vi "FileSyncLoop.vi"(5 "Name(FileSync)":string="FileSync", 7 "Protocol.lvclass":refnum<class "Protocol.lvclass">, 8 "error in":errorcluster, 11 "IniConfigFilePath":path) -> (0 "error out":errorcluster)   [LabVIEW 2014, in "FileSync -- Base.lvlib"]
uses:
  FileSync -- Base.lvlib
  Protocol/Protocol.lvclass
  Def-FileSyncConfig.ctl
  <userlib>/_NEVSTOP/JKI State Machine++/_Polymophic/Add State(s) to Queue By BOOL(Element).vi
  Global - FileSync.vi
  <userlib>/_OpenG.lib/file/file.llb/Compare Two Paths - Scalar__ogtk.vi
  ProtocolConfig/ProtocolConfig.lvclass
  <vilib>/Utility/config.llb/NI_LVConfig.lvlib
  <userlib>/_NEVSTOP/JKI State Machine++/JKI State Machine++.lvlib
panel:
  in  "Status":i32[](listbox)
  out "Statusbar":string
  out "Connected":bool
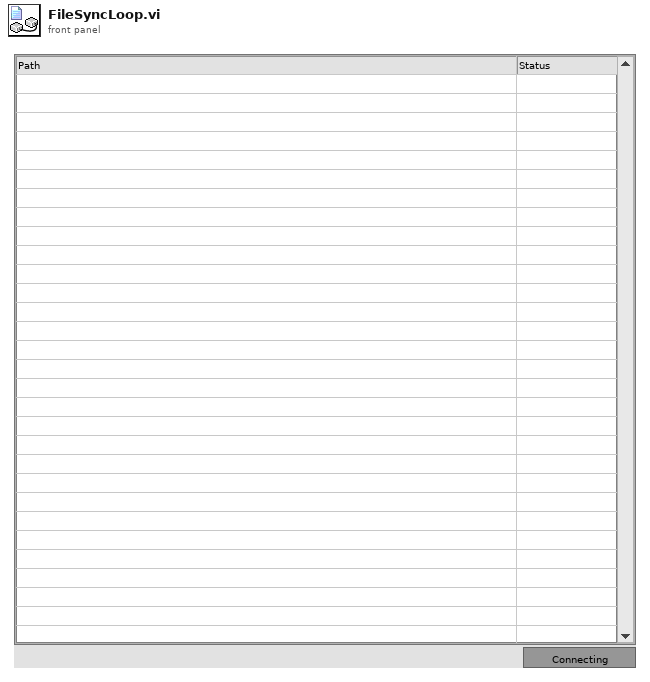
[diagram p1: front panel]
types:
  T1 = enum32{"Invalid", "Standard", "Closed", "Hidden", "Minimized", "Maximized"}
  T2 = enum32{"invalid app kind", "Development System", "Run Time System", "Student Edition", "Embedded LabVIEW", "Evaluation", "Custom"}
  T3 = typedef "FileSync -- Base.lvlib/Def-FileSyncConfig.ctl" = cluster{"Enable":bool, "DataFolder":path, "BackupFolder":path}
  T4 = cluster{"Core":cluster{"Current VI Reference":refnum<vi>, "Close Panel on Exit?":bool}, "FileSync Configuration":T3, "FileSync Status":cluster{"Connected":bool}, "Upload List":path[], "Status":refnum<vi>, "Temp:UploadingFile":path}
  T5 = cluster{"Current VI Reference":refnum<vi>, "Close Panel on Exit?":bool}
  T6 = typedef "NI_LVConfig.lvlib/Config Data RefNum.ctl" = refnum<k1>
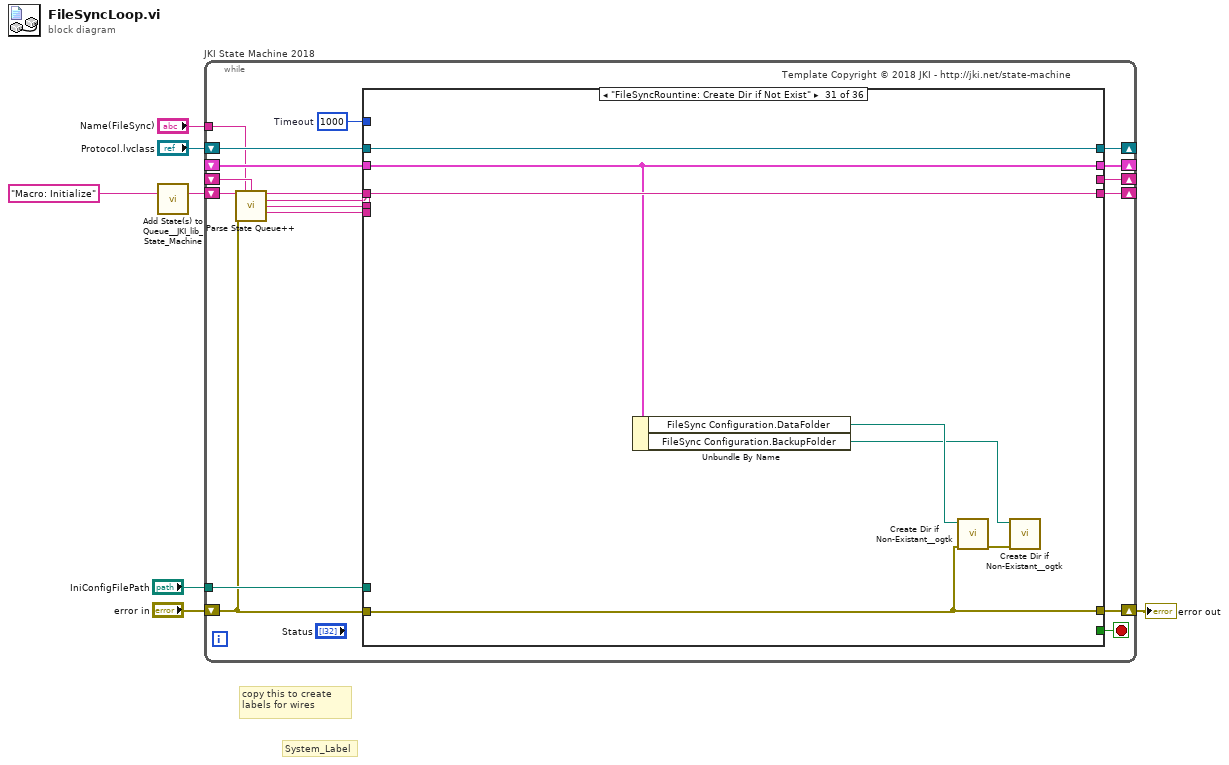
[diagram p0: block diagram]
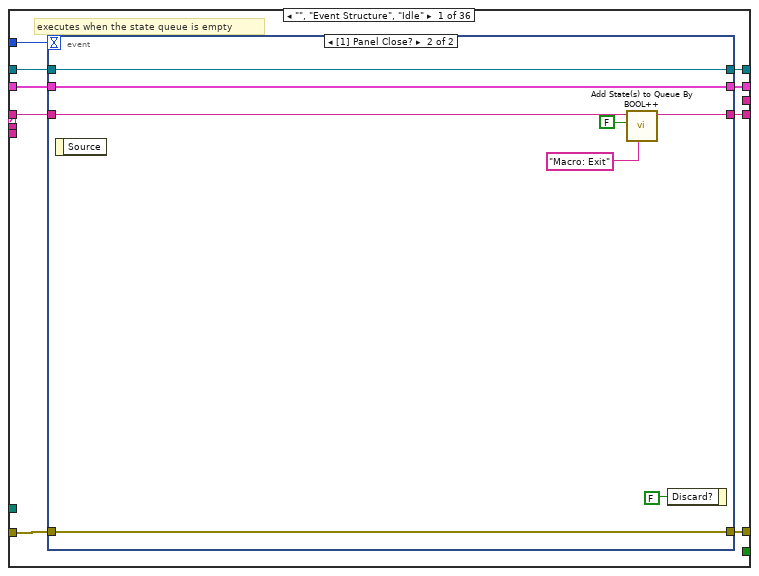
[diagram p2: hidden frame]
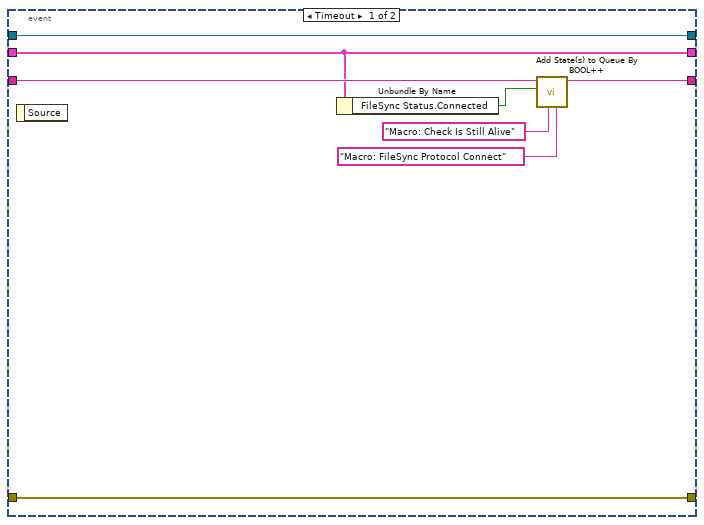
[diagram p3: hidden frame]
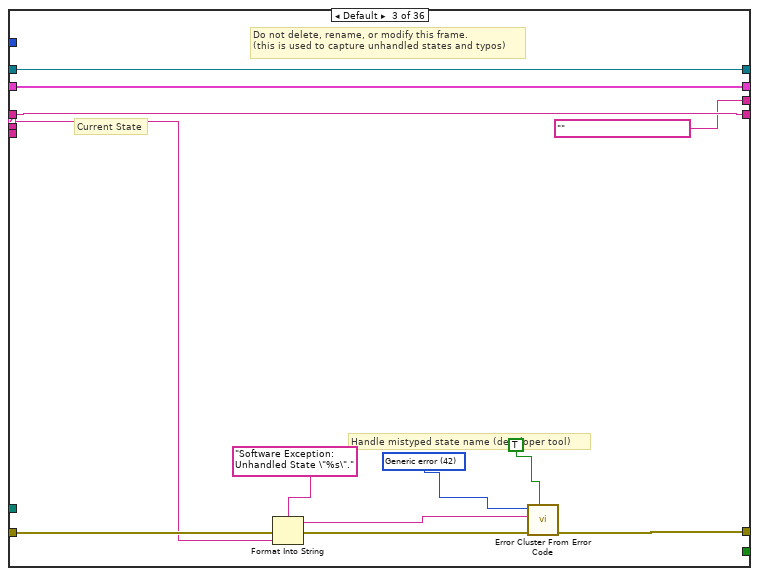
[diagram p5: hidden frame]
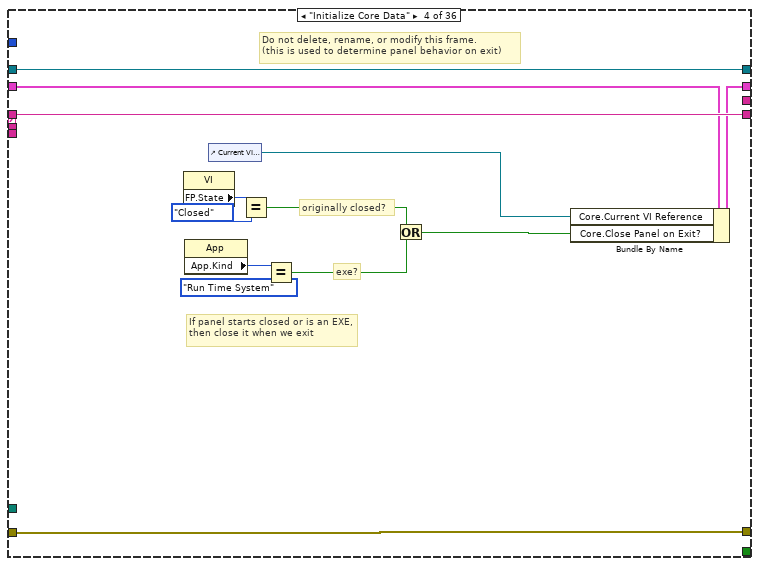
[diagram p6: hidden frame]
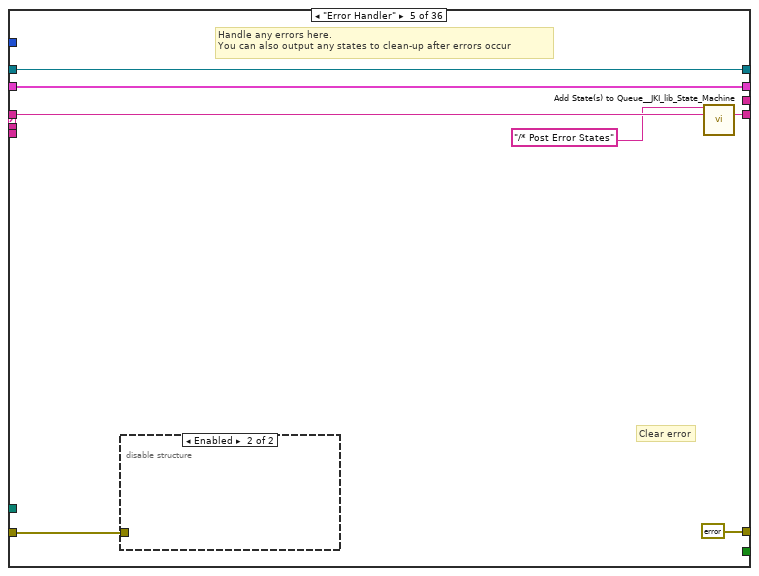
[diagram p7: hidden frame]
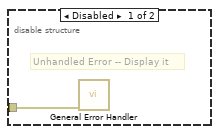
[diagram p8: hidden frame]
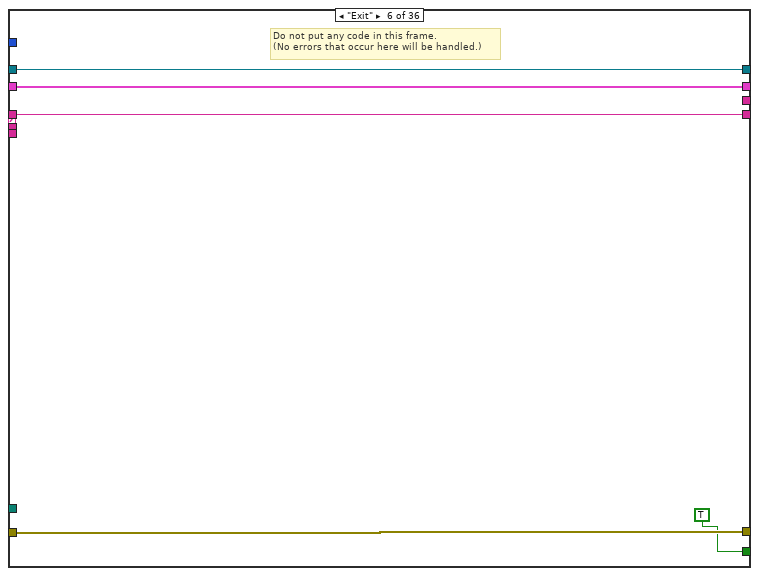
[diagram p9: hidden frame]
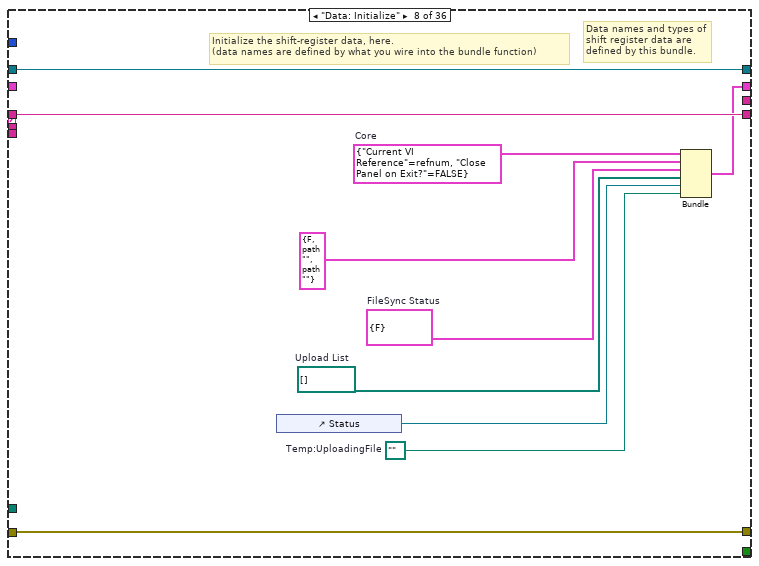
[diagram p11: hidden frame]
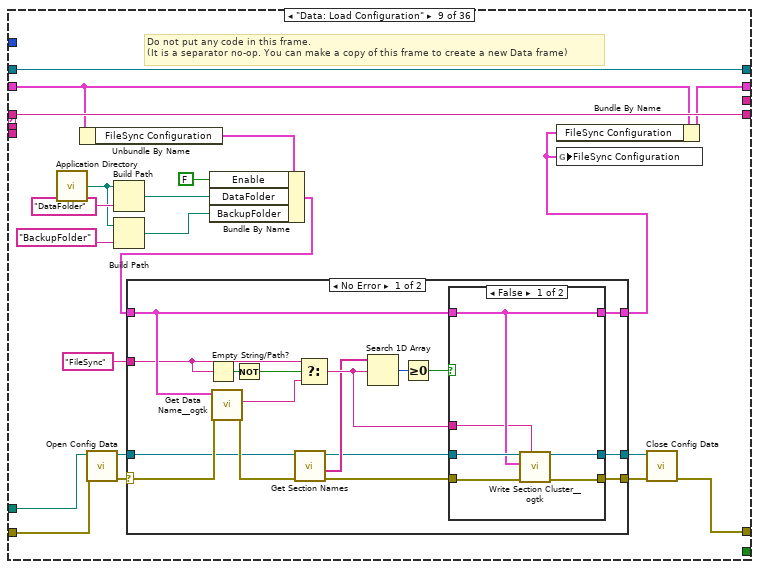
[diagram p12: hidden frame]
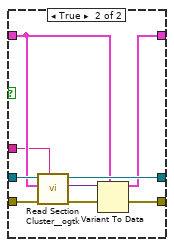
[diagram p13: hidden frame]
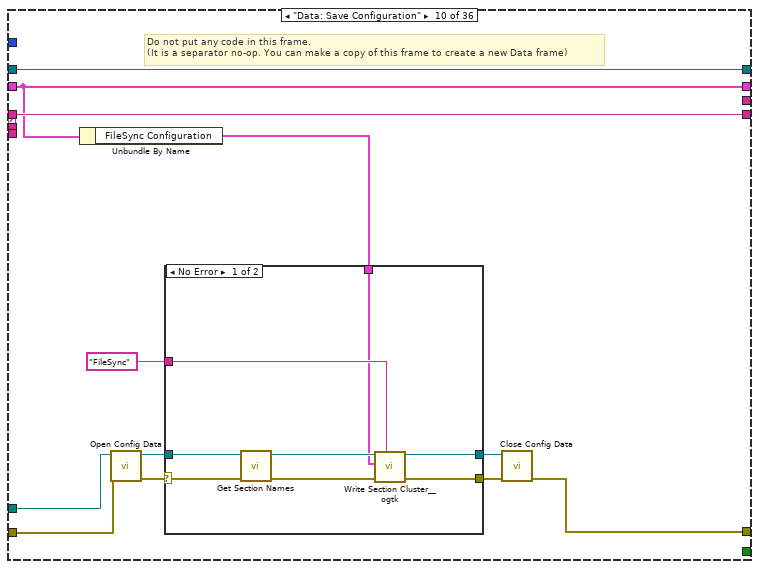
[diagram p15: hidden frame]
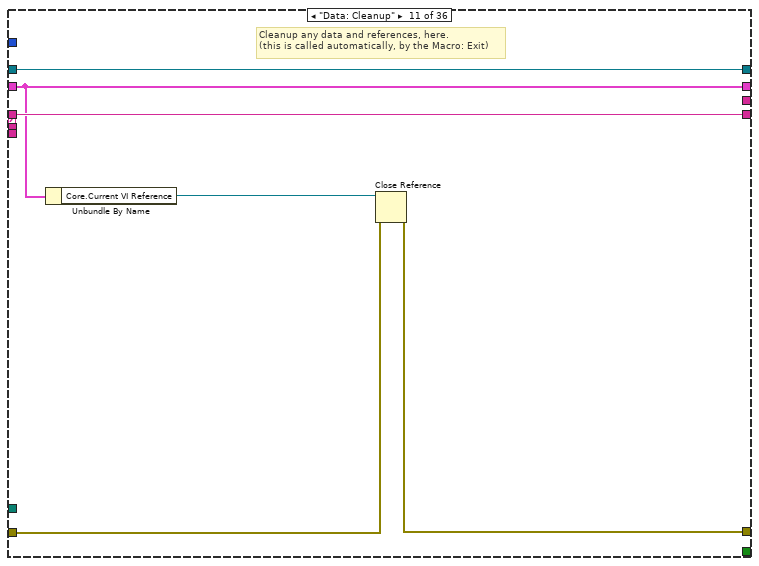
[diagram p17: hidden frame]
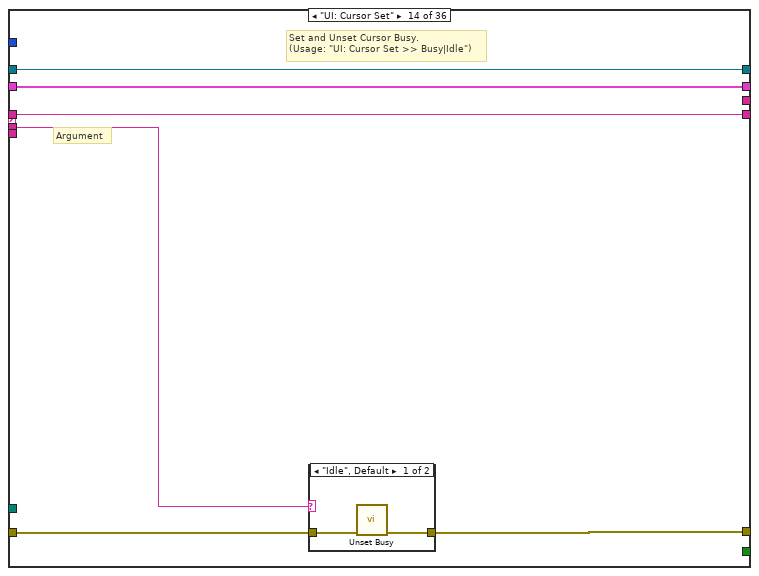
[diagram p20: hidden frame]
diagram:
  # "copy this to create labels for wires"
  # "System_Label"
  n1 = call <vilib>:"Add State(s) to Queue__JKI_lib_State_Machine.vi"("State(s) in (\"\")"="Macro: Initialize") -> ("States Out"=w7:string)  [unwired: 14 in]
  n2 = while "JKI State Machine 2018" {
    shift-right: [w22] -> _
    shift-left: _ -> [w21]
    shift-right: [w25] -> w4
    shift-left: "error in" -> [w15]
    shift-right: [w24] -> _
    shift-left: w7 -> [w16]
    shift-right: [w18] -> _
    shift-left: "Protocol.lvclass" -> [w19]
    tunnel: "IniConfigFilePath" -> [w17]
    shift-right: [w10] -> _
    shift-left: _ -> [w11]
    tunnel: "Name(FileSync)" -> [w9]
    stop <- w23 stop-if-true
    w20 = 1000  # Timeout
    # "Template Copyright © 2018 JKI - http://jki.net/state-machine"
    n3 = call <userlib>:"Parse State Queue++.vi"("State Queue"=w16, "Name(\"\" to use uuid)"=w9, "Response Arguments"=w11, "Error In (no error)"=w15) -> ("Remaining States"=w14:string, "Current State"=w12:string, "Arguments"=w13:string, "Argument - State"=w8:string)  [unwired: 6 in, 2 out]
    n4 = case shown="\"FileSyncRountine: Create Dir if Not Exist\"" w12 {
      selector: w12 -> [_ _ w57 _ _ _ _ _ _ _ _ _ _ _ _ _ _ _ _ _ _ _ _ _ _ _ _ _ _ _ _ _ _ _ _ _]
      tunnel: w14 -> [w34 w54 w60 w79 w86 w92 w96 w106 w127 w174 w190 w194 w198 w204 w215 w292 w296 w302 w306 w313 w319 w326 w341 w345 w352 w360 w371 w380 w386 w390 w397 w405 w422 w431 w441 w471]
      tunnel: w13 -> [_ _ _ _ _ _ _ _ _ _ _ _ _ w200 w210 _ _ _ _ _ _ _ _ _ _ _ _ _ _ _ _ _ _ w430 w434 w465]
      tunnel: w21 -> [w32 w52 w59 w73 w83 w91 w94 _ w118 w166 w186 w192 w197 w203 w212 w285 w294 w299 w304 w311 w317 w324 w338 w343 w351 w359 w362 w379 w385 w388 w394 w403 w418 w425 w438 w467]
      tunnel: [w31 w53 w62 w77 errorcluster {"status"=FALSE, "code"=0, "source"=""} ("error out") w90 w95 w104 w117 w165 w187 w193 w196 w201 w213 w290 w295 w300 w308 w315 w321 w328 w339 w344 w349 w355 w368 w377 w383 w389 w391 w401 w420 w427 w435 w468] -> w25
      tunnel: w15 -> [w30 w53 w61 w77 w82 w90 w95 w104 w116 w164 w188 w193 w196 w202 w214 w290 w295 w300 w308 w315 w321 w328 w339 w344 w350 w356 w369 w378 w384 w389 w391 w400 w420 w428 w439 w469]
      tunnel: [w33 w54 w60 w79 w85 w92 w96 w106 w127 w174 w190 w194 w198 w204 w215 w292 w296 w301 w307 w314 w320 w327 w340 w345 w352 w360 w370 w380 w386 w390 w397 w405 w421 w431 w441 w471] -> w24
      tunnel: [_ _ _ _ _ TRUE _ _ _ _ _ _ _ _ _ _ _ _ _ _ _ _ _ _ _ _ _ _ _ _ _ _ _ _ _ _] -> w23
      tunnel: [w29 w52 w59 w78 w83 w91 w94 w105 w119 w166 w186 w192 w197 w203 w212 w285 w294 w299 w304 w311 w317 w324 w338 w343 w351 w354 w362 w374 w385 w388 w394 w399 w417 w425 w438 w467] -> w22
      tunnel: w20 -> [w28 _ _ _ _ _ _ _ _ _ _ _ _ _ _ _ _ _ _ _ _ _ _ _ _ _ _ _ _ _ _ _ _ _ _ _]
      tunnel: w19 -> [w27 w51 w56 w67 w80 w88 w93 w102 w126 w173 w185 w191 w195 w199 w209 w291 w293 w297 w309 w316 w322 w329 w331 w342 w348 w358 w367 w376 w382 w387 w396 w404 w419 w423 w440 w470]
      tunnel: [w26 w51 w56 w67 w80 w88 w93 w102 w126 w173 w185 w191 w195 w199 w209 w289 w293 w297 w309 w316 w322 w329 w331 w342 w347 w357 w366 w375 w381 w387 w396 w404 w419 w429 w440 w470] -> w18
      tunnel: w17 -> [_ _ _ _ _ _ _ _ w120 w167 _ _ _ _ _ _ _ _ _ _ _ _ _ _ w346 _ _ _ _ _ _ _ _ _ _ _]
      tunnel: [_ _ "" ("message") _ _ _ _ _ _ _ _ _ _ _ _ _ _ _ _ _ _ _ _ _ _ _ _ _ _ _ _ _ _ _ _ _] -> w10
      tunnel: w8 -> [_ _ _ _ _ _ _ _ _ _ _ _ _ _ _ _ _ _ _ _ _ _ _ _ _ _ _ _ _ _ _ _ _ _ _ _]
      frame "", "Event Structure", "Idle" {
        # "executes when the state queue is empty"
        n5 = event shown="[1] Panel Close?" {
          selector: _ -> [_ _]
          dyn-events: _ -> [_ _]
          timeout: w28 -> [_ _]
          tunnel: w34 -> [w42 w46]
          tunnel: [w36 w50] -> w33
          tunnel: w32 -> [w39 w48]
          tunnel: [w41 w49] -> w31
          tunnel: w30 -> [w41 w49]
          tunnel: [w39 w48] -> w29
          tunnel: w27 -> [w40 w47]
          tunnel: [w40 w47] -> w26
          event Timeout {
            n6 = event-data() -> ()  [unwired: 1 in, 1 out]
            n7 = Unbundle By Name(w39) -> ("FileSync Status.Connected"=w35:bool)
            n8 = call-poly <userlib>:"Add State(s) to Queue By BOOL++.vi"("False(Empty)"="Macro: FileSync Protocol Connect" ("State(s) in Front (\"\")"), "TRUE(Empty)"="Macro: Check Is Still Alive" ("State(s) in Front (\"\")"), "Bool"=w35, "Remaining States"=w42) -> ("States Out"=w36:string)  [unwired: 7 in]
          }
          event Panel Close? {
            n9 = event-data() -> ()  [unwired: 1 in, 1 out]
            n10 = call-poly <userlib>:"Add State(s) to Queue By BOOL++.vi"("TRUE(Empty)"="Macro: Exit", "Bool"=FALSE, "Remaining States"=w46) -> ("States Out"=w50:string)  [unwired: 8 in]
            n11 = event-data("Discard?"=FALSE) -> ()  [unwired: 1 in, 1 out]
          }
        }
      }
      frame "---------- Core ----------" {
        # "Do not put any code in this frame.\n(it is a separator no-op)"
      }
      frame Default {
        w65 = 42 items=["No error", "Argument error", "Memory is full", "Out of zone", "End of file", "File already open", "Generic file I/O error", "File not found", "File permission error", "Disk is full", "Duplicate path", "Too many files open", "System feature not enabled", "Resource file not found", "Cannot add resource", "Resource not found", "Image not found", "Image memory error", "Pen does not exist", "Config type invalid", "Config token not found", "Config parse error", "Config memory error", "Bad external code format", "Bad external code offset", "External code not present", "Null window", "Destroy window error", "Null menu", "Print aborted", "Bad print record", "Print driver error", "Windows error during printing", "Memory error during printing", "Print dialog error", "Generic print error", "Invalid device refnum", "Device not found", "Device parameter error", "Device unit error", "Cannot open device", "Device call aborted", "Generic error", "Cancelled by user", "Object ID too low", "Object ID too high", "Object not in heap", "Unknown heap", "Unknown object (invalid DefProc)", "Unknown object (DefProc not in table)", "Message out of range", "Invalid (null) method", "Unknown message", "Manager call not supported", "Bad address", "Network operation in progress", "Network operation timed out", "Connection is busy", "Network attribute not supported", "Network error", "Address in use", "System out of memory", "Connection aborted", "Connection refused", "Not connected", "Already connected", "Connection closed", "Initialization error (interapplication manager)", "Bad occurrence", "Wait on unbound occurrence handler", "Occurrence queue overflow", "Datalog type conflict", "Unused", "Unrecognized type (interapplication manager)", "Memory corrupt", "Failed to make temporary DLL", "Old CIN version", "Drag socket not found", "Failed to load drop-object", "Failed to register OLE object", "Failed to release OLE object", "Format specifier type mismatch", "Unknown format specifier", "Too few format specifiers", "Too many format specifiers", "Scan failed", "Newer CIN version", "Error converting to variant", "Runtime menu error", "Password tampered", "Variant attribute not found", "Incompatible variant data type", "Event data is not available", "Event Store is not present", "Occurrence is not found", "Event Queue is not created", "Event info is not available", "Refnum passed is NULL", "Error retrieving Class GUID", "Error retrieving CoClass GUID", "Error retrieving TypeLib GUID.", "Bad built application magic bytes.", "Specific driver is different from the specific driver associated with the Logical Name.", "There is no session opened to the class driver.", "Max Error", "MAX - Error with config objects", "MAX - Error loading configuration", "MAX - Group not supported"]
        # "Current State"
        # "Do not delete, rename, or modify this frame.\n(this is used to capture unhandled states and typos)"
        # "Handle mistyped state name (developer tool)"
        n12 = Format Into String(format string="Software Exception: Unhandled State \"%s\"." ("message"), error in=w61, w57) -> (resulting string=w64:string, error out=w63:errorcluster)  [unwired: 1 in]
        n13 = call <vilib>:"Error Cluster From Error Code.vi"("show call chain? (False)"=TRUE, "error in (no error)"=w63, "error message (\"\")"=w64, "error code (0)"=w65) -> ("error out"=w62:errorcluster)  [unwired: 5 in]
      }
      frame "Initialize Core Data" {
        # "Do not delete, rename, or modify this frame.\n(this is used to determine panel behavior on exit)"
        # "originally closed?"
        # "exe?"
        # "If panel starts closed or is an EXE, then close it when we exit"
        n14 = property class="VI"() -> ("FP.State"=w70:T1)  [unwired: 2 in, 2 out]
        n15 = property class="App"() -> ("App.Kind"=w76:T2)  [unwired: 2 in, 2 out]
        n16 = control-ref of="Current VI Reference"() -> (w71:refnum<vi>)
        n17 = Equal?(x=w70, y=T1."Closed" ("Front Panel Window:State")) -> (x = y?=w68:bool)
        n18 = Equal?(x=w76, y=T2."Run Time System" ("Application:Kind")) -> (x = y?=w74:bool)
        n19 = Or(x=w68, y=w74) -> (x .or. y?=w72:bool)
        n20 = Bundle By Name(cluster=w73, "Core.Current VI Reference"=w71, "Core.Close Panel on Exit?"=w72) -> (w78:T4)
      }
      frame "Error Handler" {
        # "Handle any errors here.\nYou can also output any states to clean-up after errors occur"
        # "Clear error"
        n21 = disable-structure shown="Enabled" {
          disable-tunnel: w82 -> [w87 _]
          frame Disabled {
            # "Unhandled Error -- Display it"
            n22 = call <vilib>:"General Error Handler.vi"("error in (no error)"=w87) -> ()  [unwired: 10 in, 5 out]
          }
          frame Enabled {
          }
        }
        n23 = call <vilib>:"Add State(s) to Queue__JKI_lib_State_Machine.vi"("State(s) in Front (\"\")"="/* Post Error States", "State(s) in (\"\")"=w86) -> ("States Out"=w85:string)  [unwired: 13 in]
      }
      frame "Exit" {
        # "Do not put any code in this frame.\n(No errors that occur here will be handled.)"
      }
      frame "---------- Data ----------" {
        # "Do not put any code in this frame.\n(It is a separator no-op. You can make a copy of this frame to create a new Data frame)"
      }
      frame "Data: Initialize" {
        w97 = path ""  # Temp:UploadingFile
        w98 = path[] []  # Upload List
        w99 = cluster{"Connected":bool} {"Connected"=FALSE}  # FileSync Status
        w103 = T5 {"Current VI Reference"=refnum, "Close Panel on Exit?"=FALSE}  # Core
        # "Data names and types of shift register data are defined by this bundle."
        # "Initialize the shift-register data, here.\n(data names are defined by what you wire into the bundle function)"
        n24 = control-ref of="Status"() -> (w101:refnum<vi>)
        n25 = Bundle("Core"=w103, "FileSync Configuration"=T3 {"Enable"=FALSE, "DataFolder"=path "", "BackupFolder"=path ""}, "FileSync Status"=w99, "Upload List"=w98, "Status"=w101, "Temp:UploadingFile"=w97) -> (w105:T4)  [unwired: 1 in]
      }
      frame "Data: Load Configuration" {
        # "Do not put any code in this frame.\n(It is a separator no-op. You can make a copy of this frame to create a new Data frame)"
        n26 = call <vilib>:"Application Directory.vi"() -> ("Application Directory"=w110:path)
        n27 = Unbundle By Name(w118) -> ("FileSync Configuration"=w115:T3)
        n28 = call <vilib>:"Open Config Data.vi"("error in (no error)"=w116, "configuration file path"=w120) -> ("error out"=w124:errorcluster, "refnum"=w125:T6)  [unwired: 7 in, 1 out]
        n29 = Build Path(base path=w110, name or relative path="DataFolder") -> (appended path=w108:path)
        n30 = Build Path(base path=w110, name or relative path="BackupFolder") -> (appended path=w109:path)
        n31 = Bundle By Name(cluster=w115, "Enable"=FALSE, "DataFolder"=w108, "BackupFolder"=w109) -> (w113:T3)
        n32 = case shown="No Error" w124 {
          selector: w124 -> [w142 w160]
          tunnel: w113 -> [w141 w162]
          tunnel: "FileSync" ("section") -> [w139 _]
          tunnel: w125 -> [w131 w161]
          tunnel: [w130 w160] -> w122
          tunnel: [w129 w161] -> w123
          tunnel: [w128 w162] -> w107
          frame No Error {
            n33 = Empty String/Path?(string/path=w139) -> (empty?=w137:bool)
            n34 = call <userlib>:"Get Data Name__ogtk.vi"("error in (no error)"=w142, "Data"=w141) -> ("error out"=w143:errorcluster, "Data Name"=w140:string)  [unwired: 7 in, 1 out]
            n35 = Not(x=w137) -> (.not. x?=w138:bool)
            n36 = call <vilib>:"Get Section Names.vi"("error in (no error)"=w143, "refnum"=w131) -> ("error out"=w133:errorcluster, "section names"=w134:string[], "refnum out"=w132:T6)  [unwired: 7 in]
            n37 = Select(t=w139, s=w138, f=w140) -> (s? t:f=w144:string)
            n38 = Search 1D Array(1D array=w134, element=w144) -> (index of element=w135:i32)  [unwired: 1 in]
            n39 = Greater Or Equal To 0?(x=w135) -> (x >= 0?=w136:bool)
            n40 = case shown="False" w136 {
              tunnel: w132 -> [w150 w159]
              tunnel: [w149 w158] -> w129
              tunnel: w133 -> [w147 w157]
              tunnel: [w148 w155] -> w130
              tunnel: w141 -> [w146 w153]
              tunnel: [w146 w154] -> w128
              tunnel: w144 -> [w145 w152]
              frame False {
                n41 = call <userlib>:"Write Section Cluster__ogtk.vi"("section (optional)"=w145, "error in (no error)"=w147, "Section Formatted Cluster"=w146, "refnum"=w150) -> ("error out"=w148:errorcluster, "dup refnum"=w149:T6)  [unwired: 6 in]
              }
              frame True {
                n42 = call <userlib>:"Read Section Cluster__ogtk.vi"("section (optional)"=w152, "error in (no error)"=w157, "Section Formatted Cluster Type"=w153, "refnum"=w159) -> ("error out"=w156:errorcluster, "Section Formatted Cluster"=w151:variant, "dup refnum"=w158:T6)  [unwired: 3 in, 2 out]
                n43 = Variant To Data(error in=w156, type=w153, Variant=w151) -> (data=w154:T3, error out=w155:errorcluster)
              }
            }
          }
          frame Error {
          }
        }
        n44 = Bundle By Name(cluster=w118, "FileSync Configuration"=w107) -> (w119:T4)
        n45 = global write "Global - FileSync.vi" "FileSync Configuration"(w107) -> ()
        n46 = call <vilib>:"Close Config Data.vi"("error in (no error)"=w122, "refnum"=w123) -> ("error out"=w117:errorcluster)  [unwired: 8 in, 1 out]
      }
      frame "Data: Save Configuration" {
        # "Do not put any code in this frame.\n(It is a separator no-op. You can make a copy of this frame to create a new Data frame)"
        n47 = Unbundle By Name(w166) -> ("FileSync Configuration"=w163:T3)
        n48 = call <vilib>:"Open Config Data.vi"("error in (no error)"=w164, "configuration file path"=w167) -> ("error out"=w171:errorcluster, "refnum"=w172:T6)  [unwired: 7 in, 1 out]
        n49 = case shown="No Error" w171 {
          selector: w171 -> [w175 w183]
          tunnel: "FileSync" ("section") -> [w177 _]
          tunnel: w172 -> [w180 w184]
          tunnel: [w179 w183] -> w169
          tunnel: [w178 w184] -> w170
          tunnel: w163 -> [w176 _]
          frame No Error {
            n50 = call <vilib>:"Get Section Names.vi"("error in (no error)"=w175, "refnum"=w180) -> ("error out"=w182:errorcluster, "refnum out"=w181:T6)  [unwired: 7 in, 1 out]
            n51 = call <userlib>:"Write Section Cluster__ogtk.vi"("section (optional)"=w177, "error in (no error)"=w182, "Section Formatted Cluster"=w176, "refnum"=w181) -> ("error out"=w179:errorcluster, "dup refnum"=w178:T6)  [unwired: 6 in]
          }
          frame Error {
          }
        }
        n52 = call <vilib>:"Close Config Data.vi"("error in (no error)"=w169, "refnum"=w170) -> ("error out"=w165:errorcluster)  [unwired: 8 in, 1 out]
      }
      frame "Data: Cleanup" {
        # "Cleanup any data and references, here.\n(this is called automatically, by the Macro: Exit)"
        n53 = Unbundle By Name(w186) -> ("Core.Current VI Reference"=w189:refnum<vi>)
        n54 = Close Reference(reference=w189, error in (no error)=w188) -> (error out=w187:errorcluster)
      }
      frame "---------- UI ----------" {
        # "Do not put any code in this frame.\n(It is a separator no-op. You can make a copy of this frame to create a new UI frame)"
      }
      frame "UI: Initialize" {
      }
      frame "UI: Cursor Set" {
        # "Argument"
        # "Set and Unset Cursor Busy.\n(Usage: \"UI: Cursor Set >> Busy|Idle\")"
        n55 = case shown="\"Idle\", Default" w200 {
          tunnel: w202 -> [w206 w208]
          tunnel: [w205 w207] -> w201
          frame "Idle", Default {
            n56 = call <vilib>:"Unset Busy.vi"("error in (no error)"=w206) -> ("error out"=w205:errorcluster)  [unwired: 10 in]
          }
          frame "Busy" {
            n57 = call <vilib>:"Set Busy.vi"("error in (no error)"=w208) -> ("error out"=w207:errorcluster)  [unwired: 9 in, 1 out]
          }
        }
      }
      frame "UI: Front Panel State" {
        # "Argument"
        # "Set Front Panel Open or Closed\n(Usage: \"UI: Front Panel State >> Open|Close\")"
        n58 = Unbundle By Name(w212) -> ("Core.Current VI Reference"=w211:refnum<vi>)
        n59 = case shown="\"Open\", \"Standard\", Default" w210 {
          tunnel: w214 -> [w221 w236 w247 w260 w273]
          tunnel: [w223 w237 w249 w262 w275] -> w213
          tunnel: w211 -> [w222 w234 w248 w261 w274]
          frame "Open", "Standard", Default {
            w216 = T1."Standard" ("State")
            n60 = property class="VI"(reference=w222, error in=w221) -> (reference out=w219:refnum<vi>, error out=w220:errorcluster, "FP.State"=w218:T1)
            n61 = Not Equal?(x=w218, y=w216) -> (x != y?=w217:bool)
            n62 = case shown="True" w217 {
              tunnel: [w227 w229] -> w223
              tunnel: w220 -> [w226 w229]
              tunnel: w219 -> [w225 _]
              tunnel: w216 -> [w224 _]
              frame True {
                n63 = invoke class="VI" method="FP.Open"(reference=w225, error in=w226, "Activate"=TRUE, "State"=w224) -> (error out=w227:errorcluster)  [unwired: 1 in, 4 out]
              }
              frame False {
              }
            }
          }
          frame "Close", "Closed" {
            n64 = property class="VI"(reference=w234, error in=w236) -> (reference out=w233:refnum<vi>, error out=w235:errorcluster, "FP.State"=w231:T1)
            n65 = Not Equal?(x=w231, y=T1."Closed" ("Front Panel Window:State")) -> (x != y?=w230:bool)
            n66 = case shown="True" w230 {
              tunnel: [w238 w241] -> w237
              tunnel: w235 -> [w238 w240]
              tunnel: w233 -> [_ w239]
              frame False {
              }
              frame True {
                n67 = invoke class="VI" method="FP.Close"(reference=w239, error in=w240) -> (error out=w241:errorcluster)  [unwired: 1 in, 2 out]
              }
            }
          }
          frame "Hidden", "Hide" {
            w242 = T1."Hidden" ("State")
            n68 = property class="VI"(reference=w248, error in=w247) -> (reference out=w245:refnum<vi>, error out=w246:errorcluster, "FP.State"=w244:T1)
            n69 = Not Equal?(x=w244, y=w242) -> (x != y?=w243:bool)
            n70 = case shown="True" w243 {
              tunnel: [w253 w254] -> w249
              tunnel: w246 -> [w252 w254]
              tunnel: w245 -> [w251 _]
              tunnel: w242 -> [w250 _]
              frame True {
                n71 = invoke class="VI" method="FP.Open"(reference=w251, error in=w252, "State"=w250) -> (error out=w253:errorcluster)  [unwired: 2 in, 4 out]
              }
              frame False {
              }
            }
          }
          frame "Minimize", "Minimized" {
            w255 = T1."Minimized" ("State")
            n72 = property class="VI"(reference=w261, error in=w260) -> (reference out=w258:refnum<vi>, error out=w259:errorcluster, "FP.State"=w257:T1)
            n73 = Not Equal?(x=w257, y=w255) -> (x != y?=w256:bool)
            n74 = case shown="True" w256 {
              tunnel: [w266 w267] -> w262
              tunnel: w259 -> [w265 w267]
              tunnel: w258 -> [w264 _]
              tunnel: w255 -> [w263 _]
              frame True {
                n75 = invoke class="VI" method="FP.Open"(reference=w264, error in=w265, "State"=w263) -> (error out=w266:errorcluster)  [unwired: 2 in, 4 out]
              }
              frame False {
              }
            }
          }
          frame "Maximize", "Maximized" {
            w268 = T1."Maximized" ("State")
            n76 = property class="VI"(reference=w274, error in=w273) -> (reference out=w271:refnum<vi>, error out=w272:errorcluster, "FP.State"=w270:T1)
            n77 = Not Equal?(x=w270, y=w268) -> (x != y?=w269:bool)
            n78 = case shown="True" w269 {
              tunnel: [w279 w280] -> w275
              tunnel: w272 -> [w278 w280]
              tunnel: w271 -> [w277 _]
              tunnel: w268 -> [w276 _]
              frame True {
                n79 = invoke class="VI" method="FP.Open"(reference=w277, error in=w278, "State"=w276) -> (error out=w279:errorcluster)  [unwired: 2 in, 4 out]
              }
              frame False {
              }
            }
          }
        }
      }
      frame "UI: Update" {
        n80 = Unbundle By Name(w285) -> ("Status"=w283:refnum<vi>, "FileSync Status.Connected"=w284:bool, "Upload List"=w282:path[], "Temp:UploadingFile"=w281:path)
        "Connected" <- w284
        n81 = property class="Protocol.lvclass"(reference=w291) -> (reference out=w289:refnum<class "Protocol.lvclass">, "Properties:ProtocolConfig.lvclass"=w288:refnum<class "ProtocolConfig.lvclass">)  [unwired: 1 in, 1 out]
        n82 = call-dynamic "FlattenToDisplayString.vi"("ProtocolConfig in"=w288) -> ("String"=→"Statusbar":string)  [unwired: 8 in, 2 out]
        n83 = call "Prepare Status Table.vi"("MulticolumnListbox in"=w283, "Temp:UploadingFile"=w281, "Upload List"=w282) -> ("Array"=w286:string[][])  [unwired: 8 in]
        n84 = global write "Global - FileSync.vi" "Connected"(w284) -> ()
        n85 = property on="Status" class="MCListbox (strict)"("ItemNames"=w286) -> ()  [unwired: 2 in, 2 out]
      }
      frame "---------- Macro ----------" {
        # "Do not put any code in this frame.\n(It is a separator no-op. You can make a copy of this frame to create a new Macro frame)"
      }
      frame "Macro: Initialize" {
        # "Initialization Macro\n(This is called once, when the VI starts)"
        n86 = call <vilib>:"Add State(s) to Queue__JKI_lib_State_Machine.vi"("State(s) in Front (\"\")"="Data: Initialize\nInitialize Core Data\nData: Load Configuration\nUI: Initialize\nUI: Update\n//UI: Front Panel State >> Open\n", "State(s) in (\"\")"=w302) -> ("States Out"=w301:string)  [unwired: 13 in]
      }
      frame "Macro: FileSync Protocol Connect" {
        n87 = Unbundle By Name(w304) -> ("FileSync Configuration.Enable"=w303:bool)
        n88 = case shown="True" w303 {
          tunnel: [_ "FileSync: Load Configuration\nFileSync: Try to Connect\nUI: Update" ("State(s) in Front (\"\")")] -> w305
          frame False {
          }
          frame True {
          }
        }
        n89 = call <vilib>:"Add State(s) to Queue__JKI_lib_State_Machine.vi"("State(s) in Front (\"\")"=w305, "State(s) in (\"\")"=w306) -> ("States Out"=w307:string)  [unwired: 13 in]
      }
      frame "Macro: Check Is Still Alive" {
        n90 = call <vilib>:"Add State(s) to Queue__JKI_lib_State_Machine.vi"("State(s) in Front (\"\")"="FileSync: Check Connection is Still Alive\nUI: Update" ("State(s) in Front (\"\")"), "State(s) in (\"\")"=w313) -> ("States Out"=w314:string)  [unwired: 13 in]
      }
      frame "Macro: FileSync Routines" {
        n91 = call <vilib>:"Add State(s) to Queue__JKI_lib_State_Machine.vi"("State(s) in Front (\"\")"="FileSyncRountine: Create Dir if Not Exist\nFileSyncRountine: List Files\nFileSyncRountine: Pick Uploading File\nUI: Update" ("State(s) in Front (\"\")"), "State(s) in (\"\")"=w319) -> ("States Out"=w320:string)  [unwired: 13 in]
      }
      frame "Macro: FileSync Protocol Disconnect" {
        n92 = Unbundle By Name(w324) -> ("FileSync Status.Connected"=w323:bool)
        n93 = case shown="True" w323 {
          tunnel: [_ "FileSync: Close Connection\nFileSync: Cleanup Protocol\nUI: Update" ("State(s) in Front (\"\")")] -> w325
          frame False {
          }
          frame True {
          }
        }
        n94 = call <vilib>:"Add State(s) to Queue__JKI_lib_State_Machine.vi"("State(s) in Front (\"\")"=w325, "State(s) in (\"\")"=w326) -> ("States Out"=w327:string)  [unwired: 13 in]
      }
      frame "Macro: Exit" {
        # "Exit Macro\n(This is called once, when the VI exits)"
        n95 = Unbundle By Name(w338) -> ("Core.Close Panel on Exit?"=w337:bool)
        n96 = Select(t="UI: Front Panel State >> Close", s=w337, f="") -> (s? t:f=w334:string)
        n97 = call <vilib>:"Add State(s) to Queue__JKI_lib_State_Machine.vi"("State(s) in (\"\")"=w334, "State(s) at Back (\"\")"="Macro: FileSync Protocol Disconnect\nData: Cleanup\nExit") -> ("States Out"=w332:string)  [unwired: 13 in]
        n98 = call <vilib>:"Add State(s) to Queue__JKI_lib_State_Machine.vi"("State(s) in Front (\"\")"=w332, "State(s) in (\"\")"=w341) -> ("States Out"=w340:string)  [unwired: 13 in]
      }
      frame "---------- FileSync ----------" {
      }
      frame "FileSync: Load Configuration" {
        n99 = call-dynamic "Initialize.vi"("error in (no error)"=w350, "Path"=w346, "Protocol in"=w348) -> ("error out"=w349:errorcluster, "Protocol out"=w347:refnum<class "Protocol.lvclass">)  [unwired: 7 in]
      }
      frame "FileSync: Try to Connect" {
        n100 = call-dynamic "Connect.vi"("error in (no error)"=w356, "Protocol in"=w358) -> ("error out"=w355:errorcluster, "Connected?"=w353:bool, "Protocol out"=w357:refnum<class "Protocol.lvclass">)  [unwired: 7 in]
        n101 = Bundle By Name(cluster=w359, "FileSync Status.Connected"=w353) -> (w354:T4)
      }
      frame "FileSync: Check Connection is Still Alive" {
        n102 = call-dynamic "Check.vi"("error in (no error)"=w369, "Protocol in"=w367) -> ("error out"=w368:errorcluster, "Still alive?"=w365:bool, "Protocol out"=w366:refnum<class "Protocol.lvclass">)  [unwired: 7 in]
        n103 = Unbundle By Name(w362) -> ("FileSync Configuration.Enable"=w361:bool)
        n104 = case shown="True" w361 {
          tunnel: [_ "Macro: FileSync Routines" ("State(s) in Front (\"\")")] -> w364
          frame False {
          }
          frame True {
          }
        }
        n105 = call-poly <userlib>:"Add State(s) to Queue By BOOL++.vi"("False(Empty)"="Macro: FileSync Protocol Disconnect" ("State(s) in Front (\"\")"), "TRUE(Empty)"=w364, "Bool"=w365, "Remaining States"=w371) -> ("States Out"=w370:string)  [unwired: 7 in]
      }
      frame "FileSync: Close Connection" {
        n106 = Bundle By Name(cluster=w379, "FileSync Status.Connected"=FALSE) -> (w374:T4)
        n107 = call-dynamic "Disconnect.vi"("error in (no error)"=w378, "Protocol in"=w376) -> ("error out"=w377:errorcluster, "Protocol out"=w375:refnum<class "Protocol.lvclass">)  [unwired: 8 in]
      }
      frame "FileSync: Cleanup Protocol" {
        n108 = call-dynamic "Cleanup.vi"("error in (no error)"=w384, "Protocol in"=w382) -> ("error out"=w383:errorcluster, "Protocol out"=w381:refnum<class "Protocol.lvclass">)  [unwired: 8 in]
      }
      frame "---------- FileSyncRountine ----------" {
      }
      frame "FileSyncRountine: Create Dir if Not Exist" {
        n109 = Unbundle By Name(w394) -> ("FileSync Configuration.DataFolder"=w393:path, "FileSync Configuration.BackupFolder"=w392:path)
        n110 = call <userlib>:"Create Dir if Non-Existant__ogtk.vi"("error in (no error)"=w391, "Directory Path"=w393) -> ("error out"=w395:errorcluster)  [unwired: 7 in, 2 out]
        n111 = call <userlib>:"Create Dir if Non-Existant__ogtk.vi"("error in (no error)"=w395, "Directory Path"=w392) -> ()  [unwired: 7 in, 3 out]
      }
      frame "FileSyncRountine: List Files" {
        n112 = Unbundle By Name(w403) -> ("FileSync Configuration.DataFolder"=w402:path)
        n113 = call <vilib>:"Recursive File List.vi"("error in (no error)"=w400, "Folder Path"=w402) -> ("error out"=w401:errorcluster, "All Files in Dir"=w398:path[])  [unwired: 5 in, 3 out]
        n114 = Bundle By Name(cluster=w403, "Upload List"=w398) -> (w399:T4)
      }
      frame "FileSyncRountine: Pick Uploading File" {
        n115 = Unbundle By Name(w418) -> ("Upload List"=w407:path[])
        n116 = Index Array(array=w407) -> (element=w406:path)  [unwired: 1 in]
        n117 = Bundle By Name(cluster=w418, "Temp:UploadingFile"=w406) -> (w417:T4)
        n118 = Path To String(path=w406) -> (string=w409:string)
        n119 = Empty String/Path?(string/path=w406) -> (empty?=w416:bool)
        n120 = call <vilib>:"Build State String with Arguments__JKI_lib_State_Machine.vi"("Arguments (\"\")"=w409, "State"="FileSyncRountine: Upload" ("False(Empty)")) -> ("State with Arguments"=w408:string)  [unwired: 4 in]
        n121 = call <vilib>:"Build State String with Arguments__JKI_lib_State_Machine.vi"("Arguments (\"\")"=w409, "State"="FileSyncRountine: Move File to Backup Folder" ("False(Empty)")) -> ("State with Arguments"=w411:string)  [unwired: 4 in]
        n122 = call <vilib>:"Build State String with Arguments__JKI_lib_State_Machine.vi"("Arguments (\"\")"=w409, "State"="FileSyncRountine: Remove Empty Container Folder" ("False(Empty)")) -> ("State with Arguments"=w412:string)  [unwired: 4 in]
        n123 = call <vilib>:"Add State(s) to Queue__JKI_lib_State_Machine.vi"("State(s) in Front (\"\")"=w408, "State(s) in (\"\")"=w411, "State(s) at Back (\"\")"=w412) -> ("States Out"=w413:string)  [unwired: 12 in]
        n124 = call-poly <userlib>:"Add State(s) to Queue By BOOL++.vi"("False(Empty)"=w413, "Bool"=w416, "Remaining States"=w422) -> ("States Out"=w421:string)  [unwired: 8 in]
      }
      frame "FileSyncRountine: Upload" {
        n125 = String To Path(string=w430) -> (path=w426:path)
        n126 = Unbundle By Name(w425) -> ("FileSync Configuration.DataFolder"=w424:path)
        n127 = call-dynamic "UploadFile.vi"("Root Path"=w424, "error in (no error)"=w428, "Path"=w426, "Protocol in"=w423) -> ("error out"=w427:errorcluster, "Protocol out"=w429:refnum<class "Protocol.lvclass">)  [unwired: 6 in]
      }
      frame "FileSyncRountine: Move File to Backup Folder" {
        n128 = Unbundle By Name(w438) -> ("FileSync Configuration.BackupFolder"=w437:path, "FileSync Configuration.DataFolder"=w436:path)  [unwired: 1 out]
        n129 = String To Path(string=w434) -> (path=w433:path)
        n130 = Empty String/Path?(string/path=w433) -> (empty?=w432:bool)
        n131 = case shown="False" w432 {
          tunnel: w439 -> [w455 w462]
          tunnel: w437 -> [w453 _]
          tunnel: w436 -> [w451 _]
          tunnel: w433 -> [w442 _]
          tunnel: [w443 w462] -> w435
          frame False {
            n132 = call-poly <userlib>:"Compare Two Paths__ogtk.vi"("path2"=w442, "path1"=w451) -> ("relative path from 1 to 2"=w454:path)  [unwired: 1 in, 2 out]
            n133 = Build Path(base path=w453, name or relative path=w454) -> (appended path=w452:path)
            n134 = call <vilib>:"Check if File or Folder Exists.vi"("error in (no error)"=w455, "path"=w452) -> ("error out"=w448:errorcluster, "file or folder exists?"=w449:bool, "dup path"=w450:path)  [unwired: 7 in]
            n135 = case shown="True" w449 {
              tunnel: w450 -> [w457 w461]
              tunnel: [w457 w460] -> w447
              tunnel: w448 -> [w456 w459]
              tunnel: [w456 w458] -> w445
              frame False {
              }
              frame True {
                n136 = Delete(path (use dialog)=w461, error in=w459) -> (deleted path=w460:path, error out=w458:errorcluster)  [unwired: 3 in, 1 out]
              }
            }
            n137 = Strip Path(path=w447) -> (stripped path=w446:path)  [unwired: 1 out]
            n138 = call <userlib>:"Create Dir if Non-Existant__ogtk.vi"("error in (no error)"=w445, "Directory Path"=w446) -> ("error out"=w444:errorcluster)  [unwired: 7 in, 2 out]
            n139 = Move(source path=w442, error in=w444, 10:w447) -> (error out=w443:errorcluster)  [unwired: 2 in, 2 out]
          }
          frame True {
          }
        }
      }
      frame "FileSyncRountine: Remove Empty Container Folder" {
        n140 = Unbundle By Name(w467) -> ("FileSync Configuration.DataFolder"=w466:path)  [unwired: 1 out]
        n141 = String To Path(string=w465) -> (path=w464:path)
        n142 = Empty String/Path?(string/path=w464) -> (empty?=w463:bool)
        n143 = case shown="False" w463 {
          tunnel: w469 -> [w475 w497]
          tunnel: [w474 w497] -> w468
          tunnel: w466 -> [w473 _]
          tunnel: w464 -> [w472 _]
          frame False {
            n144 = while {
              tunnel: w473 -> [w482]
              shift-right: [w478] -> w474
              shift-left: w475 -> [w479]
              shift-right: [w477] -> _
              shift-left: w472 -> [w483]
              stop <- w476 stop-if-true
              n145 = Strip Path(path=w483) -> (stripped path=w477:path)  [unwired: 1 out]
              n146 = List Folder(path=w477, error in=w479) -> (path out=w484:path, filenames=w490:string[], folder names=w489:string[], error out=w481:errorcluster)  [unwired: 2 in]
              n147 = Empty Array?(array=w490) -> (empty?=w488:bool)
              n148 = Empty Array?(array=w489) -> (empty?=w487:bool)
              n149 = Not Equal?(x=w482, y=w477) -> (x != y?=w485:bool)
              n150 = And(x=w488, y=w487) -> (x .and. y?=w486:bool)
              n151 = And(x=w485, y=w486) -> (x .and. y?=w480:bool)
              n152 = case shown="False" w480 {
                tunnel: w484 -> [_ w496]
                tunnel: w481 -> [w492 w495]
                tunnel: [w492 w494] -> w478
                tunnel: [TRUE FALSE] -> w476
                frame False {
                }
                frame True {
                  n153 = Delete(path (use dialog)=w496, error in=w495) -> (error out=w494:errorcluster)  [unwired: 3 in, 2 out]
                }
              }
            }
          }
          frame True {
          }
        }
      }
    }
  }
  "error out" <- w4
